vi "ErrorHandling.Fglb.vi"(7 "Action":T3=enum."get", 8 "error in (no error)":errorcluster, 10 "Error in":T1, 11 "Event source":T2) -> (0 "error out":errorcluster, 1 "changed":bool, 2 "Errors out":T1[](array[typedef]))   [LabVIEW 2016]
uses:
  ErrorHandling.Fglb.Action.ctl
  EventLog/EventLog.EventSource.ctl
  CitTemplate/citTemplate.errData.ctl
panel:
  out "Errors":T1[](array[typedef])
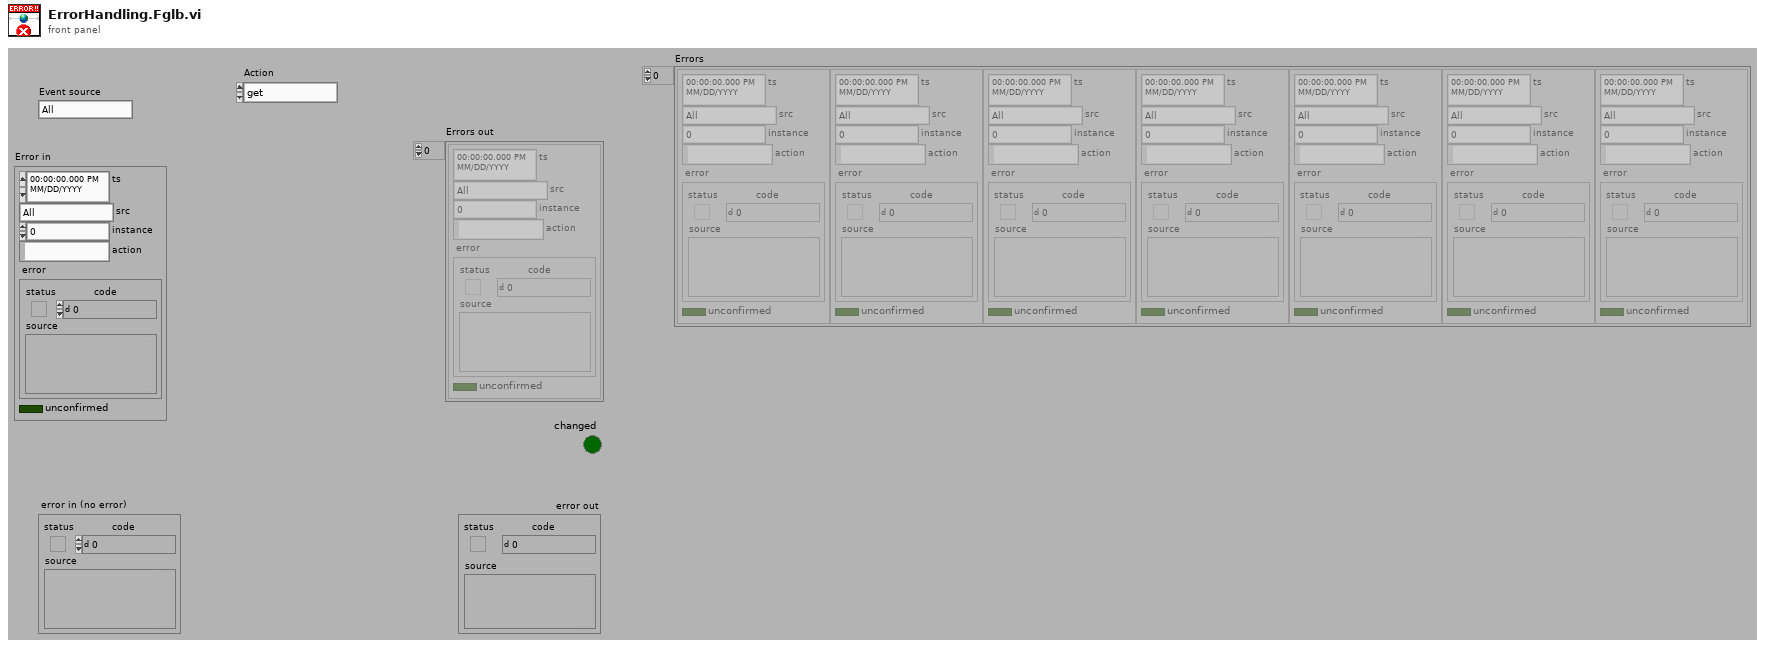
[diagram p1: front panel]
types:
  T1 = typedef "citTemplate.errData.ctl" = cluster{"ts":timestamp, "src":T2, "instance":i32, "action":string, "error":errorcluster, "unconfirmed":bool}
  T2 = typedef "EventLog.EventSource.ctl" = enum16{"All", "Gui", "Ref", "File", "Arch", "Seq", "CPX", "DB", "Laser", "Scan.P", "Scan.O", "PLC"}
  T3 = typedef "ErrorHandling.Fglb.Action.ctl" = enum16{"init", "add", "clear", "confirm", "check", "get"}
  T4 = cluster{"src":T2, "instance":i32, "action":string}
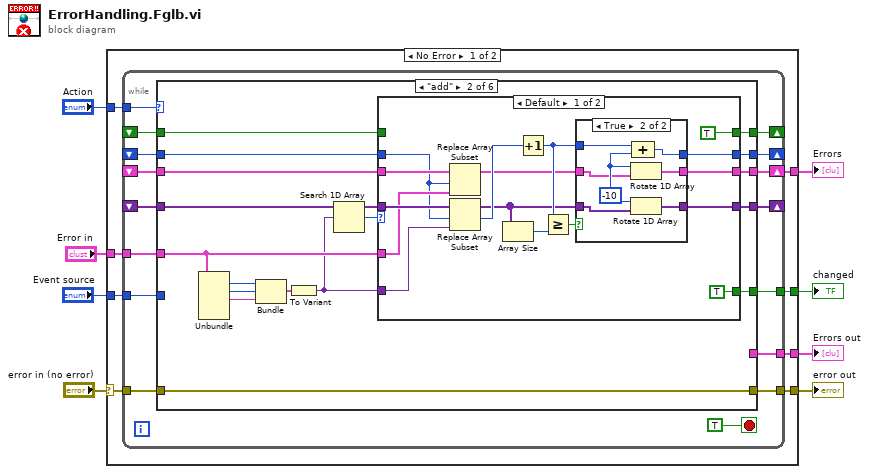
[diagram p0: block diagram]
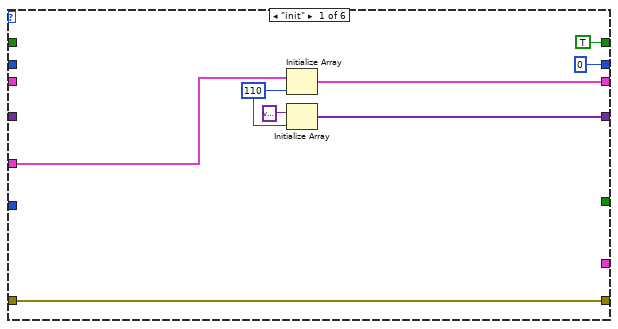
[diagram p2: hidden frame]
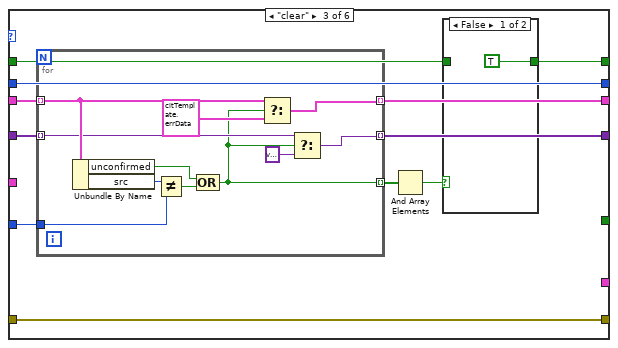
[diagram p5: hidden frame]
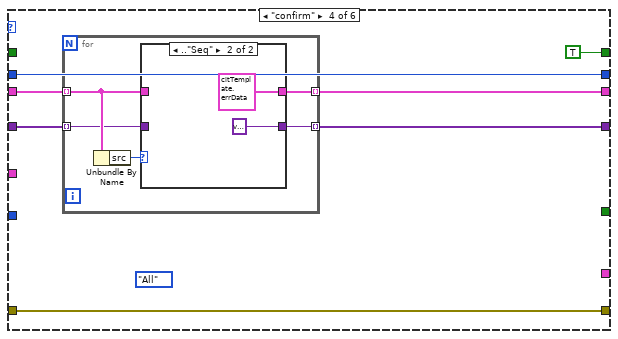
[diagram p7: hidden frame]
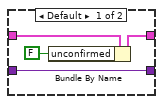
[diagram p8: hidden frame]
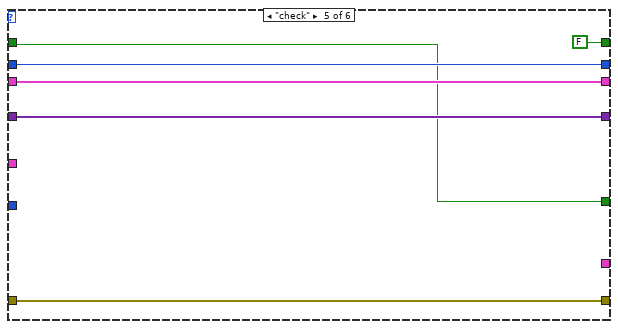
[diagram p9: hidden frame]
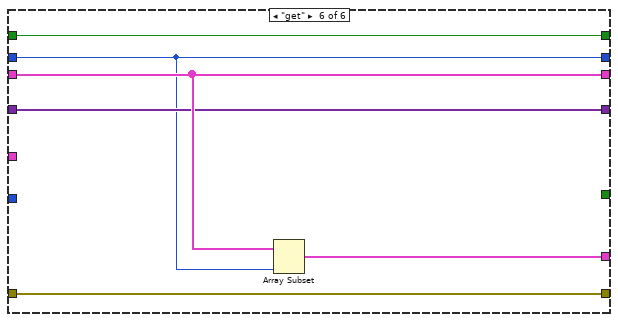
[diagram p10: hidden frame]
diagram:
  n1 = case shown="No Error" "error in (no error)" {
    selector: "error in (no error)" -> [w16 w141]
    tunnel: [w13 w141] -> w7
    tunnel: "Action" -> [w15 _]
    tunnel: "Error in" -> [w14 _]
    tunnel: "Event source" -> [w12 _]
    tunnel: [w11 _] -> w4
    tunnel: [w10 _] -> w3
    tunnel: [w9 _] -> w1
    frame No Error {
      n2 = while {
        tunnel: w16 -> [w27]
        tunnel: w15 -> [w32]
        tunnel: w14 -> [w31]
        shift-right: [w30] -> w10
        shift-left: _ -> [w29]
        tunnel: [w26] -> w13
        tunnel: w12 -> [w25]
        shift-right: [w24] -> _
        shift-left: _ -> [w23]
        tunnel: [w22] -> w11
        shift-right: [w21] -> _
        shift-left: _ -> [w20]
        shift-right: [w19] -> _
        shift-left: _ -> [w18]
        tunnel: [w17] -> w9
        stop <- TRUE stop-if-true
        n3 = case shown="\"add\"" w32 {
          tunnel: w31 -> [w40 w46 _ _ _ _]
          tunnel: [w38 w57 w97 w117 w131 w138] -> w30
          tunnel: w29 -> [_ w55 w96 w116 w131 w138]
          tunnel: w27 -> [w39 w56 w95 w115 w134 w140]
          tunnel: [w39 w56 w95 w115 w134 w140] -> w26
          tunnel: w25 -> [_ _ w94 _ _ _]
          tunnel: [TRUE w54 w87 TRUE FALSE w139] -> w24
          tunnel: w23 -> [_ w53 w90 _ w129 w139]
          tunnel: [_ _ _ _ _ w137] -> w22
          tunnel: [w34 w44 w91 w112 w132 w136] -> w21
          tunnel: w20 -> [_ w45 w92 w113 w132 w136]
          tunnel: [0 w48 w93 w111 w130 w135] -> w19
          tunnel: w18 -> [_ w49 w93 w111 w130 w135]
          tunnel: [_ w42 _ _ w129 _] -> w17
          frame "init" {
            w36 = 110 ("dimension size")
            n4 = Initialize Array(w40, w36) -> (w38:T1[])
            n5 = Initialize Array(variant ("variant"), w36) -> (w34:variant[])
          }
          frame "add" {
            n6 = Unbundle(w46) -> ("src"=w52:T2, "instance"=w51:i32, "action"=w41:string)  [unwired: 3 out]
            n7 = Bundle("src"=w52, "instance"=w51, "action"=w41) -> (w50:T4)  [unwired: 1 in]
            n8 = To Variant(anything=w50) -> (Variant=w43:variant)
            n9 = Search 1D Array(1D array=w45, element=w43) -> (index of element=w47:i32)  [unwired: 1 in]
            n10 = case shown="Default" w47 {
              tunnel: [w60 w86] -> w57
              tunnel: w55 -> [w69 w86]
              tunnel: [TRUE w85] -> w54
              tunnel: w53 -> [_ w85]
              tunnel: w49 -> [w64 w84]
              tunnel: [w59 w84] -> w48
              tunnel: w46 -> [w70 _]
              tunnel: w45 -> [w71 w83]
              tunnel: [w62 w83] -> w44
              tunnel: w43 -> [w65 _]
              tunnel: [TRUE _] -> w42
              frame Default {
                n11 = Replace Array Subset(array=w69, new element=w70, index=w64) -> (w61:T1[])
                n12 = Replace Array Subset(array=w71, new element=w65, index=w64) -> (w63:variant[])
                n13 = Array Size(array=w63) -> (size(s)=w68:i32)
                n14 = Increment(x=w64) -> (x+1=w66:i32)
                n15 = Greater Or Equal?(x=w66, y=w68) -> (x >= y?=w67:bool)
                n16 = case shown="True" w67 {
                  tunnel: w66 -> [w74 w82]
                  tunnel: w63 -> [w73 w76]
                  tunnel: [w73 w81] -> w62
                  tunnel: [w74 w80] -> w59
                  tunnel: w61 -> [w75 w77]
                  tunnel: [w75 w79] -> w60
                  frame False {
                  }
                  frame True {
                    w78 = -10 ("y")
                    n17 = Rotate 1D Array(1:w77, 2:w78) -> (0:w79:T1[])
                    n18 = Rotate 1D Array(1:w76, 2:w78) -> (0:w81:variant[])
                    n19 = Compound Arithmetic op=ADD(w82, w78) -> (w80:i32)
                  }
                }
              }
              frame 0.. {
              }
            }
          }
          frame "clear" {
            n20 = for {
              tunnel: [w106] -> w97 mode=indexing
              tunnel: w96 -> [w107] mode=indexing
              tunnel: w94 -> [w110]
              tunnel: w92 -> [w105] mode=indexing
              tunnel: [w103] -> w91 mode=indexing
              tunnel: [w100] -> w89 mode=indexing
              n21 = Unbundle By Name(w107) -> ("unconfirmed"=w101:bool, "src"=w109:T2)
              n22 = Not Equal?(x=w109, y=w110) -> (x != y?=w104:bool)
              n23 = Compound Arithmetic op=OR(w101, w104) -> (w100:bool)
              n24 = Select(t=w107, s=w100, f=T1 {"ts"=timestamp(0 s since 1904-01-01), "src"=enum."All", "instance"=0, "action"="", "error"={"status"=FALSE, "code"=0, "source"=""}, "unconfirmed"=FALSE} ("new element/subarray")) -> (s? t:f=w106:T1)
              n25 = Select(t=w105, s=w100, f=variant) -> (s? t:f=w103:variant)
            }
            n26 = And Array Elements(Boolean array=w89) -> (logical AND=w88:bool)
            n27 = case shown="False" w88 {
              tunnel: w90 -> [_ w99]
              tunnel: [TRUE w99] -> w87
              frame False {
              }
              frame True {
              }
            }
          }
          frame "confirm" {
            (unwired) EventLog.EventSource."All" ("src")
            n28 = for {
              tunnel: [w122] -> w117 mode=indexing
              tunnel: w116 -> [w121] mode=indexing
              tunnel: w113 -> [w119] mode=indexing
              tunnel: [w118] -> w112 mode=indexing
              n29 = Unbundle By Name(w121) -> ("src"=w120:T2)
              n30 = case shown="..\"Seq\"" w120 {
                tunnel: [w125 T1 {"ts"=timestamp(0 s since 1904-01-01), "src"=enum."All", "instance"=0, "action"="", "error"={"status"=FALSE, "code"=0, "source"=""}, "unconfirmed"=FALSE} ("new element/subarray")] -> w122
                tunnel: w121 -> [w126 _]
                tunnel: w119 -> [w123 _]
                tunnel: [w123 variant ("f")] -> w118
                frame Default {
                  n31 = Bundle By Name(cluster=w126, "unconfirmed"=FALSE) -> (w125:T1)
                }
                frame .."Seq" {
                }
              }
            }
          }
          frame "check" {
          }
          frame "get" {
            n32 = Array Subset(array=w138, length=w135) -> (w137:T1[])  [unwired: 1 in]
          }
        }
      }
    }
    frame Error {
    }
  }
  "error out" <- w7
  "Errors out" <- w4
  "Errors" <- w3
  "changed" <- w1
